vi "获取版本信息.vi"(8 "error in (no error)":errorcluster caption="错误输入（无错误）", 11 "file path":path) -> (0 "error out":errorcluster caption="错误输出", 3 "版本信息":cluster{"版本号":string, "更新内容":string}[](array[cluster]))   [LabVIEW 2016, in "数据传输系统-05.lvlib" / "update.lvlib"]
uses:
  update.lvlib
  http client.lvclass
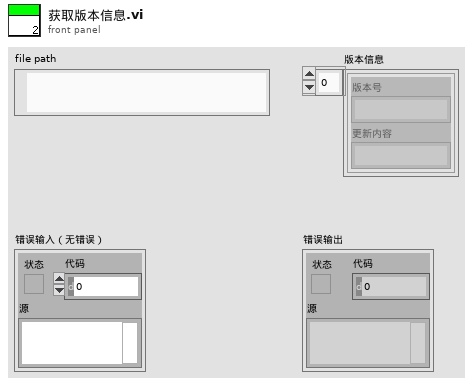
[diagram p1: front panel]
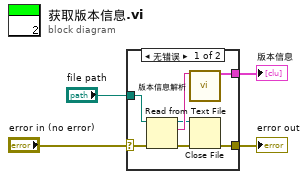
[diagram p0: block diagram]
diagram:
  n1 = case shown="无错误" "error in (no error)" {
    selector: "error in (no error)" -> [w8 w12]
    tunnel: [w5 w12] -> w3
    tunnel: [w11 _] -> w2
    tunnel: "file path" -> [w10 _]
    frame No Error {
      n2 = Read from Text File(file (use dialog)=w10, error in=w8) -> (refnum out=w6:refnum<file>, text=w9:string, error out=w7:errorcluster)  [unwired: 2 in, 1 out]
      n3 = call "版本信息解析.vi"("body"=w9) -> ("版本信息"=w11:cluster{"版本号":string, "更新内容":string}[])  [unwired: 18 in]
      n4 = Close File(refnum=w6, error in=w7) -> (error out=w5:errorcluster)  [unwired: 1 out]
    }
    frame Error {
    }
  }
  "error out" <- w3
  "版本信息" <- w2
